vi "Digital IO (178x Smart Camera).vi"() -> ()   [LabVIEW 2023]
doc: "The Digital IO (178x Smart Camera) example shows how to use the static I/O available on the ISC-178x smart camera."
uses:
  <vilib>/vision/driver/NI_Vision_Acquisition_Software.lvlib
  <resource>/objmgr/imaqdx.rc
panel:
  in  "ISO Outputs":bool[](array[boolean])=[FALSE, FALSE, FALSE, FALSE]
  in  "Stop":bool
  in  "ISO Inputs":T1(array[cluster])=[{"Status"=FALSE, "Edge Counter"=0, "Reset Counter"=FALSE}, {"Status"=FALSE, "Edge Counter"=0, "Reset Counter"=FALSE}, {"Status"=FALSE, "Edge Counter"=0, "Reset Counter"=FALSE}, {"Status"=FALSE, "Edge Counter"=0, "Reset Counter"=FALSE}]
  in  "Camera Name":refnum<k21> caption="IMAQdx Session"
  # "Overview: Demonstrates how to use the static I/O available on a ISC-178x smart camera.\nRequirements: Vision Acquisition Software, a ISC-178x smart camera.\nInstructions: \n1. Open a new LabVIEW Project by selecting Project»Create Project. Select Add this VI when prompted to add this VI to the project.\n2. Right click on the top-level project item in the tree and select New»Targets and Devices\n3. Select the ISC-178x smart camera you want to run this example with, and click OK.\n4. Drag this VI from My Computer to the smart camera target.\n5. Double click on the example under the smart camera, select the Camera Name, and run the VI."
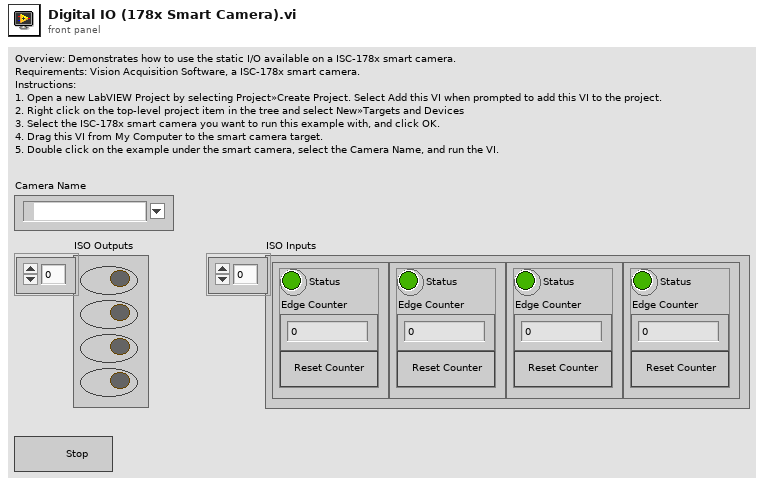
[diagram p1: front panel]
types:
  T1 = cluster{"Status":bool, "Edge Counter":u32, "Reset Counter":bool}[]
  T2 = typedef "IMAQdx.ctl" = refnum<k21>
  T3 = cluster{"Status":bool, "Edge Counter":u32, "Reset Counter":bool}
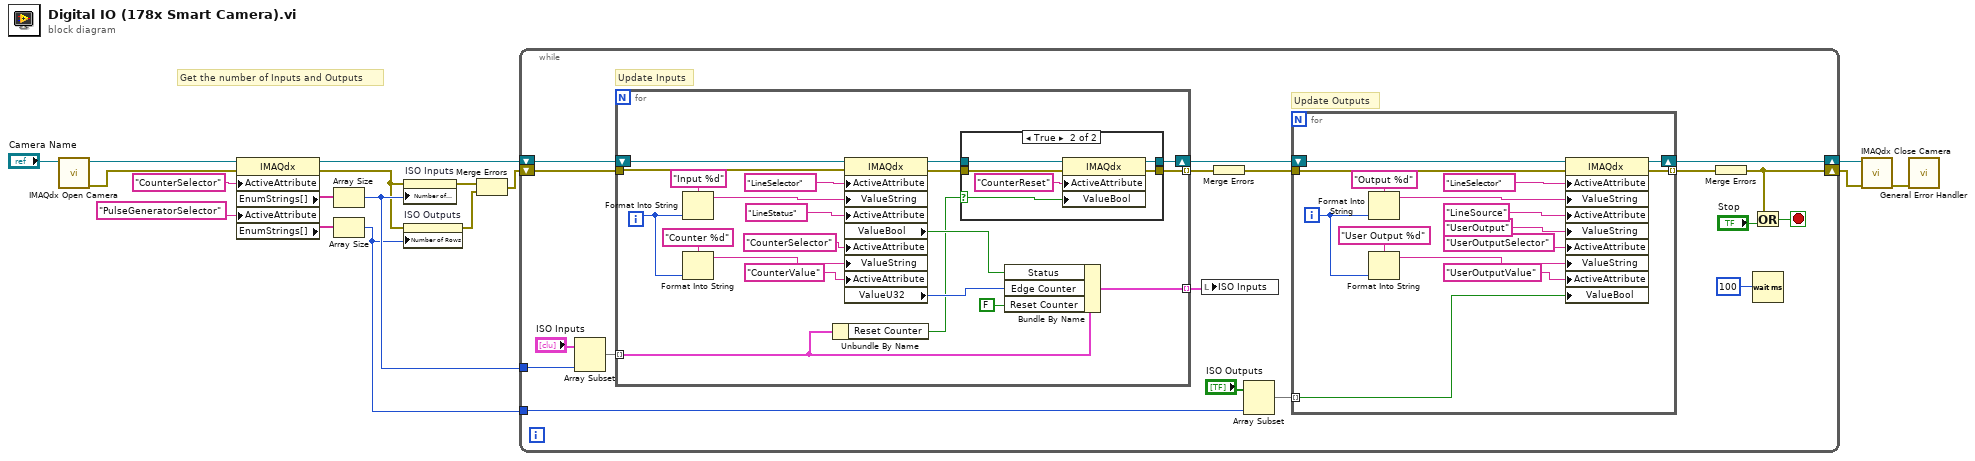
[diagram p0: block diagram]
diagram:
  # "Get the number of Inputs and Outputs"
  n1 = call <vilib>:"IMAQdx Open Camera.vi"("Session In"="Camera Name") -> ("error out"=w11:errorcluster, "Session Out"=w13:T2)  [unwired: 2 in, 7 out]
  n2 = property class="IMAQdx"(reference=w13, error in=w11, "ActiveAttribute"="CounterSelector", "ActiveAttribute"="PulseGeneratorSelector") -> (reference out=w12:T2, error out=w4:errorcluster, "EnumStrings[]"=w8:string[], "EnumStrings[]"=w7:string[])
  n3 = Array Size(array=w8) -> (size(s)=w6:i32)
  n4 = Array Size(array=w7) -> (size(s)=w5:i32)
  n5 = property on="ISO Inputs" class="Arr"(error in=w4, "Number of Columns"=w6) -> (error out=w3:errorcluster)  [unwired: 1 in, 1 out]
  n6 = property on="ISO Outputs" class="Arr (strict)"(error in=w4, "Number of Rows"=w5) -> (error out=w2:errorcluster)  [unwired: 1 in, 1 out]
  n7 = Merge Errors(w3, w2) -> (w1:errorcluster)
  n8 = while {
    shift-right: [w29] -> w15
    shift-left: w12 -> [w35]
    shift-right: [w27] -> w14
    shift-left: w1 -> [w34]
    tunnel: w6 -> [w23]
    tunnel: w5 -> [w19]
    stop <- w31 stop-if-true
    # "Update Inputs"
    # "Update Outputs"
    n9 = Array Subset(array="ISO Inputs", length=w23) -> (w21:T1)  [unwired: 1 in]
    n10 = for "Update Inputs" {
      tunnel: w21 -> [w64] mode=indexing
      tunnel: w34 -> [w65]
      tunnel: [w54] -> w25 mode=indexing
      shift-right: [w56] -> w30
      shift-left: w35 -> [w71]
      tunnel: [w60] -> w33 mode=indexing
      i -> [w51]
      n11 = Format Into String(format string="Input %d", w51) -> (resulting string=w58:string)  [unwired: 2 in, 1 out]
      n12 = Format Into String(format string="Counter %d", w51) -> (resulting string=w59:string)  [unwired: 2 in, 1 out]
      n13 = Unbundle By Name(w64) -> ("Reset Counter"=w53:bool)
      n14 = property class="IMAQdx"(reference=w71, error in=w65, "ActiveAttribute"="LineSelector", "ValueString"=w58, "ActiveAttribute"="LineStatus", "ActiveAttribute"="CounterSelector", "ValueString"=w59, "ActiveAttribute"="CounterValue") -> (reference out=w57:T2, error out=w55:errorcluster, "ValueBool"=w63:bool, "ValueU32"=w62:u32)
      n15 = case shown="True" w53 {
        selector: w53 -> [_ w74]
        tunnel: w57 -> [w73 w79]
        tunnel: [w73 w78] -> w56
        tunnel: w55 -> [w72 w77]
        tunnel: [w72 w76] -> w54
        frame False {
        }
        frame True {
          n16 = property class="IMAQdx"(reference=w79, error in=w77, "ActiveAttribute"="CounterReset", "ValueBool"=w74) -> (reference out=w78:T2, error out=w76:errorcluster)
        }
      }
      n17 = Bundle By Name(cluster=w64, "Status"=w63, "Edge Counter"=w62, "Reset Counter"=FALSE) -> (w60:T3)
    }
    n18 = local write "ISO Inputs"(w33) -> ()
    n19 = Merge Errors(w25) -> (w28:errorcluster)
    n20 = Array Subset(array="ISO Outputs", length=w19) -> (w18:bool[])  [unwired: 1 in]
    n21 = for "Update Outputs" {
      shift-right: [w49] -> w29
      shift-left: w30 -> [w50]
      tunnel: w18 -> [w36] mode=indexing
      tunnel: w28 -> [w48]
      tunnel: [w47] -> w26 mode=indexing
      i -> [w37]
      n22 = Format Into String(format string="Output %d", w37) -> (resulting string=w45:string)  [unwired: 2 in, 1 out]
      n23 = Format Into String(format string="User Output %d", w37) -> (resulting string=w39:string)  [unwired: 2 in, 1 out]
      n24 = property class="IMAQdx"(reference=w50, error in=w48, "ActiveAttribute"="LineSelector", "ValueString"=w45, "ActiveAttribute"="LineSource", "ValueString"="UserOutput" ("ActiveAttribute"), "ActiveAttribute"="UserOutputSelector", "ValueString"=w39, "ActiveAttribute"="UserOutputValue", "ValueBool"=w36) -> (reference out=w49:T2, error out=w47:errorcluster)
    }
    n25 = Merge Errors(w26) -> (w27:errorcluster)
    n26 = Or(x=w27, y="Stop") -> (x .or. y?=w31:bool)
    n27 = Wait (ms)(milliseconds to wait=u32 100 ("millisecond multiple")) -> ()  [unwired: 1 out]
  }
  n28 = call <vilib>:"IMAQdx Close Camera.vi"("error in"=w14, "Session In"=w15) -> ("error out"=w17:errorcluster)  [unwired: 9 out]
  n29 = call <vilib>:"General Error Handler.vi"("error in (no error)"=w17) -> ()  [unwired: 2 in, 13 out]
